vi "process.vi"(8 "error in (no error)":errorcluster, 11 "Subscription in":refnum<class "Subscription.lvclass">) -> ()   [LabVIEW 2013, in "MQTT Base.lvlib" / "Subscription.lvclass"]
uses:
  Subscription.lvclass
  Subscription.lvclass/Subscription.ctl
  TopicFilter/TopicFilter.lvclass/TopicFilter.ctl
  TopicFilter/TopicFilter.lvclass
  <vilib>/LabVIEW Open Source Project/MQTT Control Packets/Control Packets/PUBLISH/PUBLISH.lvclass
panel:
  out "Topic Filter":string
  out "Numeric":i32
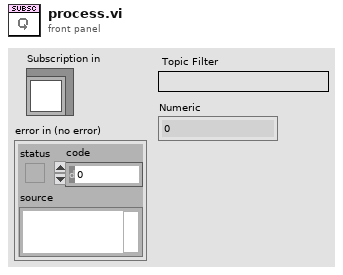
[diagram p1: front panel]
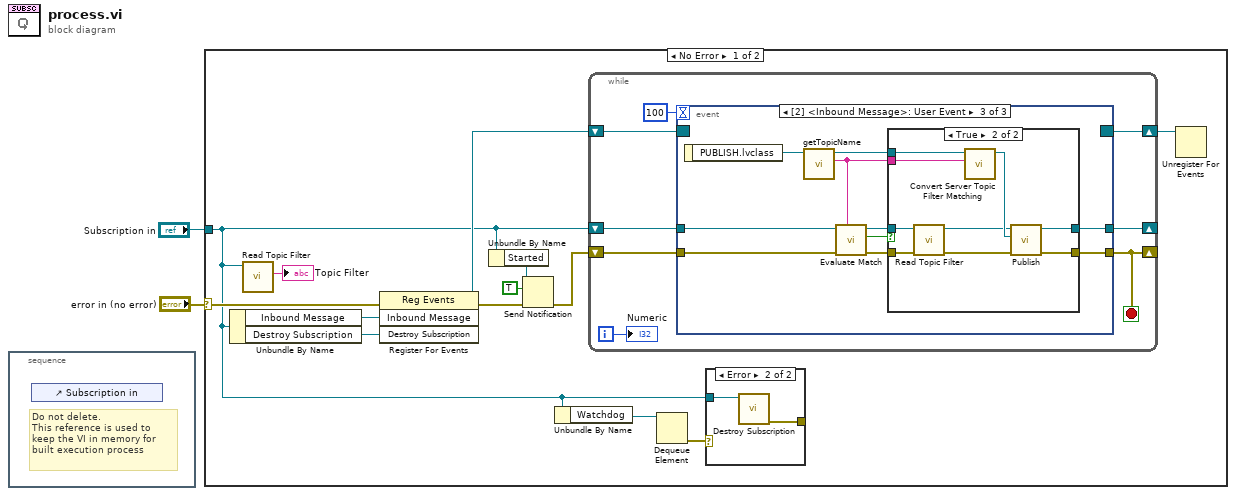
[diagram p0: block diagram]
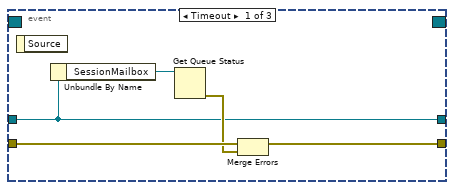
[diagram p3: hidden frame]
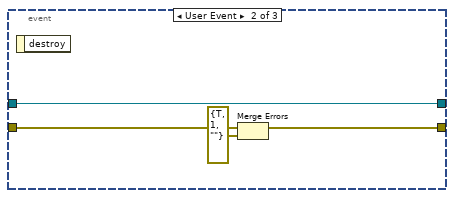
[diagram p4: hidden frame]
diagram:
  n1 = stacked-sequence {
    frame #0 {
      # "Do not delete.\nThis reference is used to keep the VI in memory for built execution process"
      n2 = control-ref of="Subscription in"() -> ()  [unwired: 1 out]
    }
  }
  n3 = case shown="No Error" "error in (no error)" {
    selector: "error in (no error)" -> [w13 _]
    tunnel: "Subscription in" -> [w3 _]
    frame No Error {
      n4 = Unbundle By Name(w3) -> ("Inbound Message"=w6:refnum<user-event>, "Destroy Subscription"=w5:refnum<user-event>)
      n5 = call "Read Topic Filter.vi"("Subscription in"=w3) -> ("Topic Filter"=→"Topic Filter":string)  [unwired: 7 in, 3 out]
      n6 = register-events(error in=w13, w6, w5) -> (reference out=w11:refnum<event-registration>, error out=w12:errorcluster)  [unwired: 1 in]
      n7 = Unbundle By Name(w3) -> ("Started"=w4:refnum<notifier>)
      n8 = Send Notification(notification=TRUE, notifier=w4, error in (no error)=w12) -> (error out=w14:errorcluster)  [unwired: 1 out]
      n9 = Unbundle By Name(w3) -> ("Watchdog"=w8:refnum<queue>)
      n10 = while {
        shift-right: [w20] -> _
        shift-left: w14 -> [w21]
        shift-right: [w23] -> w10
        shift-left: w11 -> [w24]
        shift-right: [w18] -> _
        shift-left: w3 -> [w22]
        i -> [w19]
        stop <- w20 stop-if-true
        n11 = event shown="[2] <Inbound Message>: User Event" {
          selector: w24 -> [_ _ _]
          dyn-events: [_ _ _] -> w23
          timeout: 100 -> [_ _ _]
          tunnel: w22 -> [w26 w32 w42]
          tunnel: w21 -> [w29 w34 w43]
          tunnel: [w27 w33 w44] -> w20
          tunnel: [w26 w32 w36] -> w18
          event Timeout {
            n12 = event-data() -> ()  [unwired: 1 in, 1 out]
            n13 = Unbundle By Name(w26) -> ("SessionMailbox"=w30:refnum<queue>)
            n14 = Get Queue Status(queue=w30) -> (error out=w28:errorcluster)  [unwired: 2 in, 7 out]
            n15 = Merge Errors(w29, w28) -> (w27:errorcluster)
          }
          event User Event {
            n16 = event-data() -> ()  [unwired: 1 in, 1 out]
            n17 = Merge Errors(w34, errorcluster {"status"=TRUE, "code"=1, "source"=""} ("error in")) -> (w33:errorcluster)
          }
          event User Event {
            n18 = event-data() -> ("PUBLISH.lvclass"=w41:refnum<class "PUBLISH.lvclass">)  [unwired: 1 in]
            n19 = call <vilib>:"getTopicName.vi"("PUBLISH in"=w41) -> ("Topic"=w35:string, "PUBLISH out"=w40:refnum<class "PUBLISH.lvclass">)  [unwired: 8 in, 1 out]
            n20 = call "Evaluate Match.vi"("Topic"=w35, "error in (no error)"=w43, "Subscription in"=w42) -> ("error out"=w37:errorcluster, "Matched"=w39:bool, "Subscription out"=w38:refnum<class "Subscription.lvclass">)  [unwired: 5 in, 1 out]
            n21 = case shown="True" w39 {
              tunnel: [w46 w55] -> w44
              tunnel: w37 -> [w46 w49]
              tunnel: w38 -> [w45 w51]
              tunnel: w40 -> [_ w53]
              tunnel: [w45 w54] -> w36
              tunnel: w35 -> [_ w47]
              frame False {
              }
              frame True {
                n22 = call "Read Topic Filter.vi"("error in (no error)"=w49, "Subscription in"=w51) -> ("error out"=w48:errorcluster, "Subscription out"=w50:refnum<class "Subscription.lvclass">)  [unwired: 6 in, 2 out]
                n23 = call <vilib>:"Convert Server Topic Filter Matching.vi"("Matching Topic Filter"=w47, "PUBLISH"=w53) -> ("Server PUBLISH"=w52:refnum<class "PUBLISH.lvclass">)  [unwired: 8 in, 1 out]
                n24 = call "Publish.vi"("error in (no error)"=w48, "PUBLISH"=w52, "Subscription in"=w50) -> ("error out"=w55:errorcluster, "Subscription out"=w54:refnum<class "Subscription.lvclass">)  [unwired: 7 in]
              }
            }
          }
        }
        "Numeric" <- w19
      }
      n25 = Dequeue Element(queue=w8) -> (error out=w7:errorcluster)  [unwired: 2 in, 3 out]
      n26 = case shown="Error" w7 {
        tunnel: w3 -> [_ w17]
        tunnel: [_ w16] -> _
        frame No Error {
        }
        frame Error {
          n27 = call "Destroy Subscription.vi"("Subscription in"=w17) -> ("error out"=w16:errorcluster)  [unwired: 9 in, 1 out]
        }
      }
      n28 = Unregister For Events(event registration refnum=w10) -> ()  [unwired: 1 in, 1 out]
    }
    frame Error {
    }
  }
